vi "Delete Line.vi"(8 "error in":errorcluster, 10 "Line Name":string, 11 "SQLite configuration in":refnum<class "SQLite configuration.lvclass">) -> (0 "error out":errorcluster, 2 "Deleted Line":T1, 3 "SQLite configuration out":refnum<class "SQLite configuration.lvclass">)   [LabVIEW 2014, in "SQLite configuration.lvclass"]
doc: "Deletes a line based on its name."
uses:
  SQLite configuration.lvclass
  Line.ctl
  <vilib>/NI/Tag Bus Module Framework/channel/TBM channel.lvclass
  SQLite configuration.lvclass/SQLite configuration.ctl
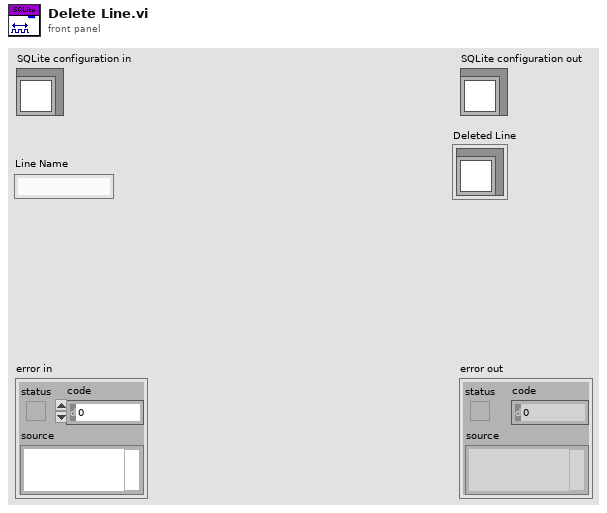
[diagram p1: front panel]
types:
  T1 = typedef "SQLite configuration.lvclass/Line.ctl" = cluster{"channel":refnum<class "TBM channel.lvclass">}
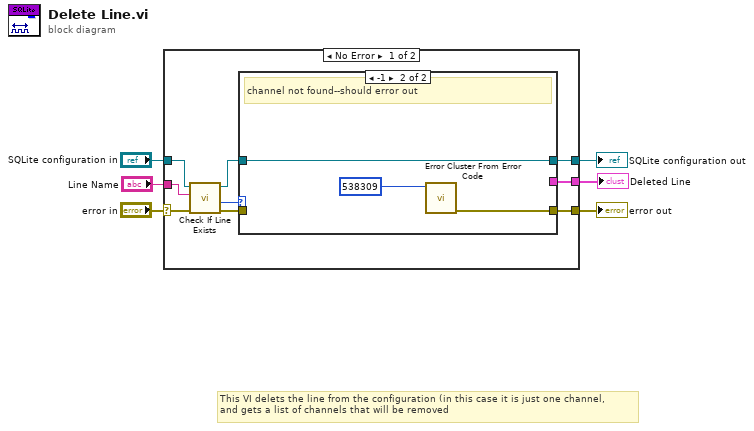
[diagram p0: block diagram]
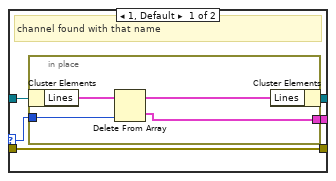
[diagram p2: hidden frame]
diagram:
  # "This VI delets the line from the configuration (in this case it is just one channel, \nand gets a list of channels that will be removed"
  n1 = case shown="No Error" "error in" {
    selector: "error in" -> [w9 w28]
    tunnel: [w15 w28] -> w6
    tunnel: [w14 w29] -> w5
    tunnel: "SQLite configuration in" -> [w12 w29]
    tunnel: "Line Name" -> [w13 _]
    tunnel: [w8 _] -> w1
    frame No Error {
      n2 = call-dynamic "Check If Line Exists.vi"("error in"=w9, "Name to Locate"=w13, "SQLite configuration in"=w12) -> ("error out"=w10:errorcluster, "Index"=w7:i32, "SQLite configuration out"=w11:refnum<class "SQLite configuration.lvclass">)  [unwired: 4 in, 2 out]
      n3 = case shown="-1" w7 {
        selector: w7 -> [w16 _]
        tunnel: [w18 w27] -> w15
        tunnel: w11 -> [w20 w25]
        tunnel: [w19 w25] -> w14
        tunnel: w10 -> [w18 _]
        tunnel: [w17 _] -> w8
        frame 1, Default {
          # "channel found with that name"
          n4 = in-place {
            in-place-border: w16 -> [w24]
            in-place-border: [w21] -> w17
            n5 = in-place-cluster #1(w20) -> ("Lines"=w23:T1[])
            n6 = Delete From Array(array=w23, index=w24) -> (deleted portion=w21:T1, array with subset deleted=w22:T1[])  [unwired: 1 in]
            n7 = in-place-cluster #1("Lines"=w22) -> (w19:refnum<class "SQLite configuration.lvclass">)
          }
        }
        frame -1 {
          # "channel not found--should error out"
          n8 = call <vilib>:"Error Cluster From Error Code.vi"("error code (0)"=538309) -> ("error out"=w27:errorcluster)  [unwired: 8 in]
        }
      }
    }
    frame Error {
    }
  }
  "error out" <- w6
  "SQLite configuration out" <- w5
  "Deleted Line" <- w1
